vi "36DUT Plot From Spread Sheet.vi"(6 "Plot":T1(ring), 7 "No of Rows":i32=10496, 8 "error in (no error)":errorcluster, 10 "Bank":i32(ring) items=["C1", "C2", "C3", "D_C1", "D_C2", "D_C3", "D_B1_C1", "D_B1_C2", "D_B1_C3"], 11 "file path (dialog if empty)":path) -> (0 "error out":errorcluster, 3 "Delta C_Min Plot":dbl[][](graph) caption="(Y) Multi Plot 2")   [LabVIEW 2012]
uses:
  <vilib>/Utility/file.llb/Read From Spreadsheet File (string).vi
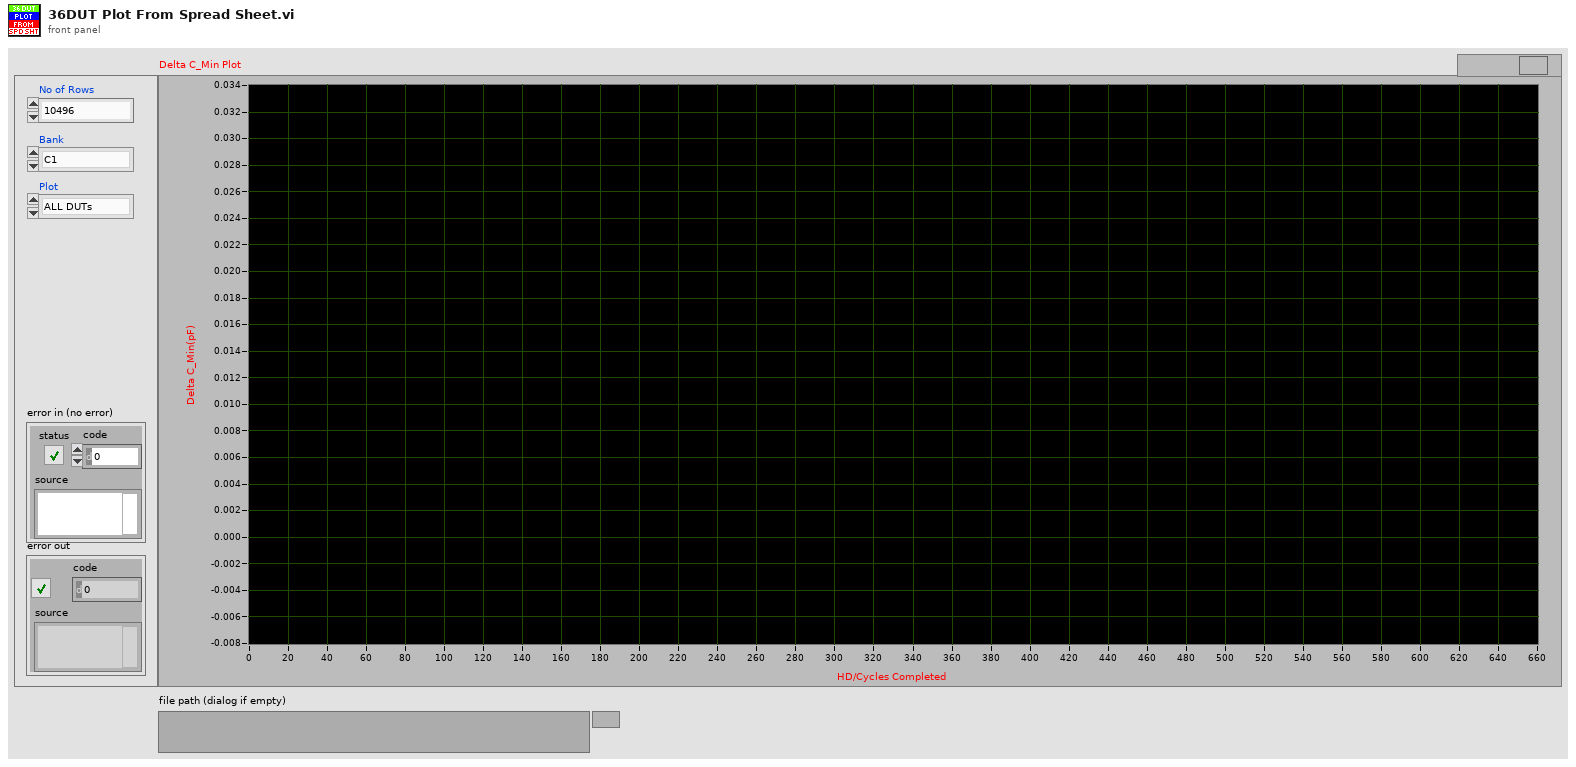
[diagram p1: front panel]
types:
  T1 = enum16{"ALL DUTs", "DUT 01", "DUT 02", "DUT 03", "DUT 04", "DUT 05", "DUT 06", "DUT 07", "DUT 08", "DUT 09", "DUT 10", "DUT 11", "DUT 12", "DUT 13", "DUT 14", "DUT 15", "DUT 16", "DUT 17", "DUT 18", "DUT 19", "DUT 20", "DUT 21", "DUT 22", "DUT 23", "DUT 24", "DUT 25", "DUT 26", "DUT 27", "DUT 28", "DUT 29", "DUT 30", "DUT 31", "DUT 32", "DUT 33", "DUT 34", "DUT 35", "DUT 36"}
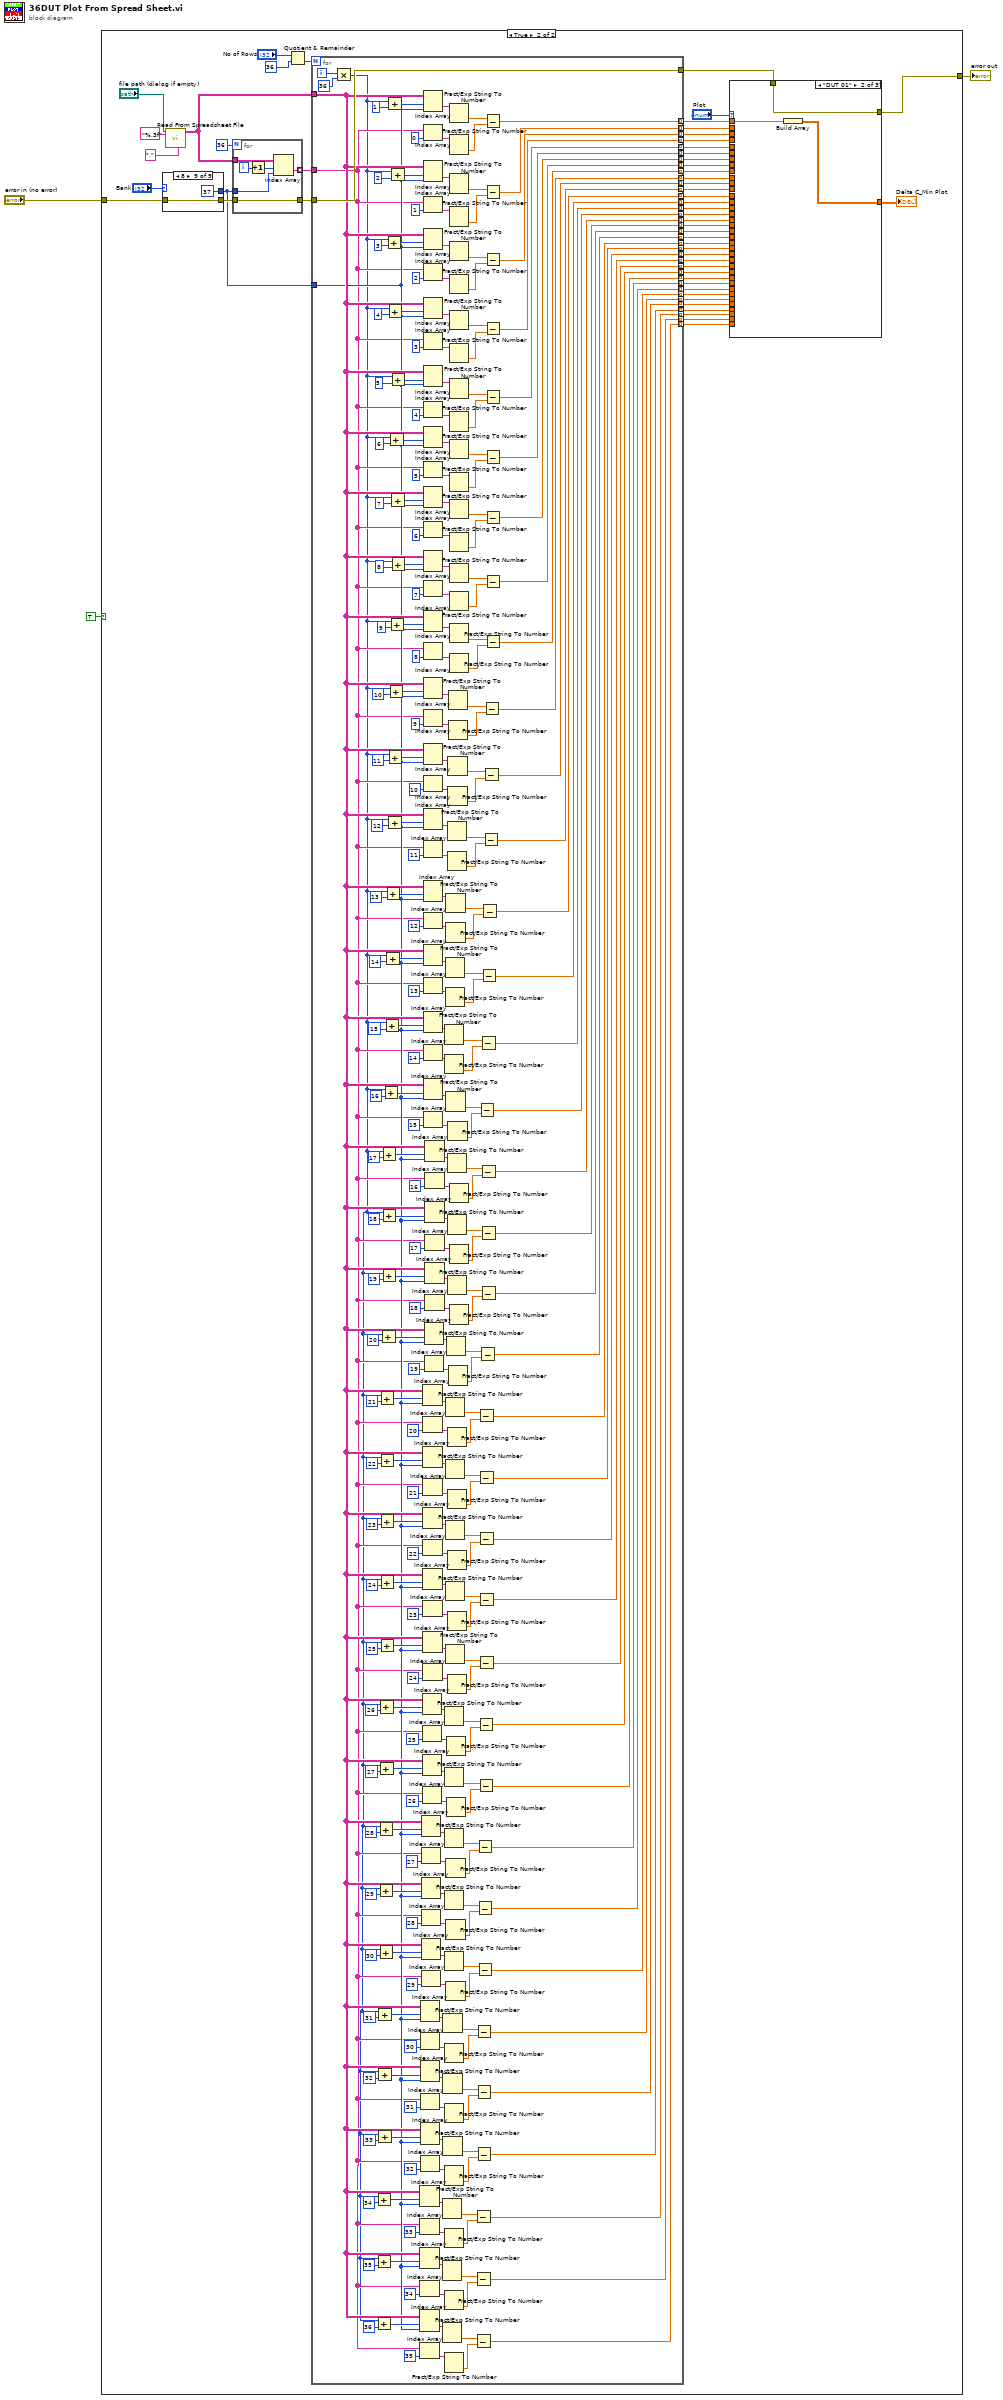
[diagram p0: block diagram]
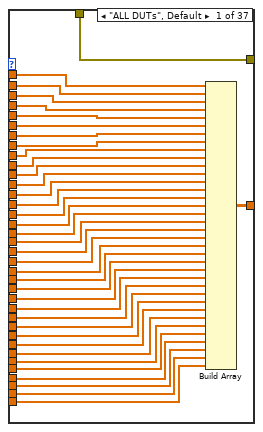
[diagram p3: hidden frame]
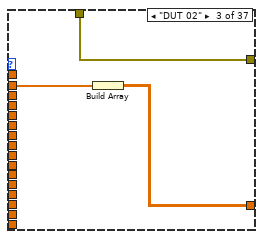
[diagram p4: hidden frame]
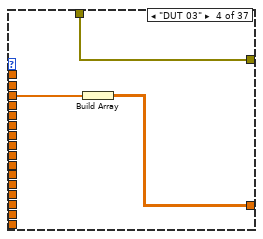
[diagram p5: hidden frame]
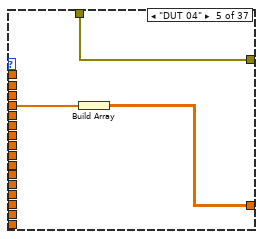
[diagram p6: hidden frame]
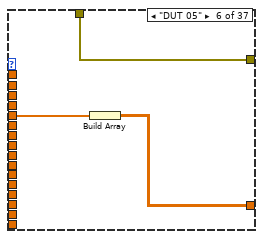
[diagram p7: hidden frame]
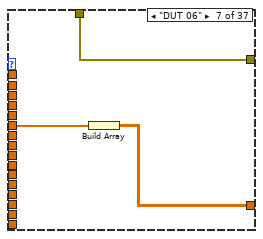
[diagram p8: hidden frame]
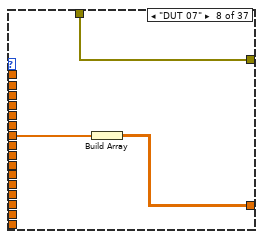
[diagram p9: hidden frame]
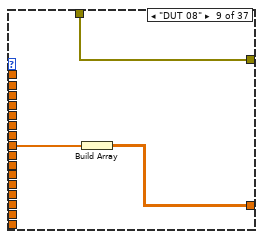
[diagram p10: hidden frame]
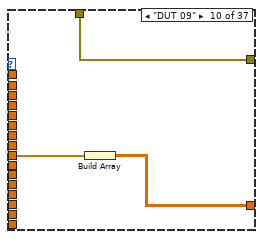
[diagram p11: hidden frame]
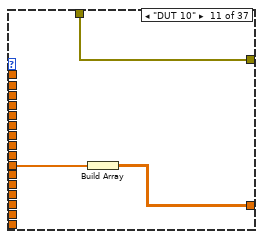
[diagram p12: hidden frame]
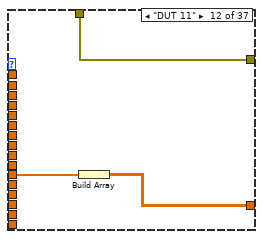
[diagram p13: hidden frame]
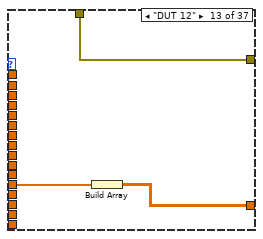
[diagram p14: hidden frame]
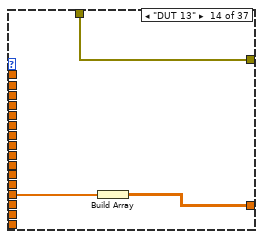
[diagram p15: hidden frame]
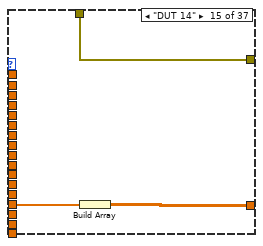
[diagram p16: hidden frame]
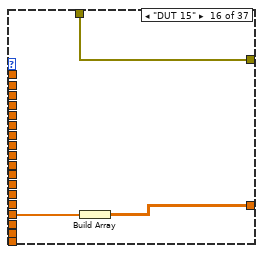
[diagram p17: hidden frame]
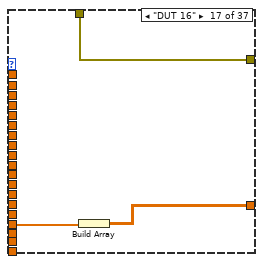
[diagram p18: hidden frame]
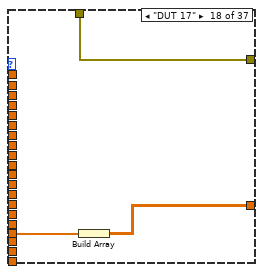
[diagram p19: hidden frame]
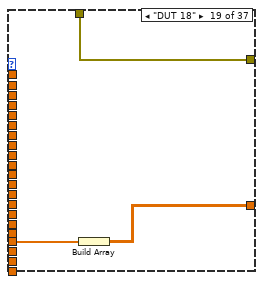
[diagram p20: hidden frame]
diagram:
  n1 = case shown="True" TRUE {
    tunnel: "error in (no error)" -> [w4 w31]
    tunnel: [w4 w25] -> w2
    frame False {
    }
    frame True {
      n2 = case shown="8" "Bank" {
        tunnel: [5 40 75 119 120 121 35 36 37] -> w27
        tunnel: [w205 w207 w209 w212 w214 w216 w217 w219 w221] -> w28
        tunnel: w31 -> [w205 w207 w209 w212 w214 w216 w217 w219 w221]
        frame 0, Default {
        }
        frame 1 {
        }
        frame 2 {
        }
        frame 3 {
        }
        frame 4 {
        }
        frame 5 {
        }
        frame 6 {
        }
        frame 7 {
        }
        frame 8 {
        }
      }
      n3 = call-poly <vilib>:"Read From Spreadsheet File.vi"("delimiter (\\t)"="," ("delimiter (\\t)"), "format (%s)"="%.3f" ("format (%.3f)"), "file path (dialog if empty)"="file path (dialog if empty)") -> ("all rows"=w55:string[][])  [unwired: 4 in, 4 out]
      n4 = for {
        N: 36 -> [_]
        tunnel: w55 -> [w523]
        tunnel: [w522] -> w54 mode=indexing
        tunnel: w27 -> [w518]
        tunnel: [w519] -> w30
        tunnel: w28 -> [w519]
        i -> [w521]
        n5 = Increment(x=w521) -> (x+1=w520:i32)
        n6 = Index Array(array=w523, index (row)=w520, index (col)=w518) -> (element=w522:string)
      }
      n7 = Quotient & Remainder(x="No of Rows", y=36) -> (floor(x/y)=w50:i32)  [unwired: 1 out]
      n8 = for {
        N: w50 -> [_]
        tunnel: w55 -> [w246]
        tunnel: w54 -> [w244]
        tunnel: [w404] -> w48 mode=indexing
        tunnel: [w403] -> w47 mode=indexing
        tunnel: [w402] -> w46 mode=indexing
        tunnel: [w401] -> w45 mode=indexing
        tunnel: [w400] -> w44 mode=indexing
        tunnel: [w399] -> w43 mode=indexing
        tunnel: [w398] -> w42 mode=indexing
        tunnel: [w397] -> w41 mode=indexing
        tunnel: [w396] -> w40 mode=indexing
        tunnel: [w395] -> w39 mode=indexing
        tunnel: [w394] -> w38 mode=indexing
        tunnel: [w393] -> w37 mode=indexing
        tunnel: [w392] -> w36 mode=indexing
        tunnel: [w391] -> w35 mode=indexing
        tunnel: [w390] -> w34 mode=indexing
        tunnel: [w389] -> w33 mode=indexing
        tunnel: w30 -> [w388]
        tunnel: [w388] -> w29
        tunnel: w27 -> [w245]
        tunnel: [w243] -> w24 mode=indexing
        tunnel: [w242] -> w23 mode=indexing
        tunnel: [w241] -> w22 mode=indexing
        tunnel: [w240] -> w21 mode=indexing
        tunnel: [w239] -> w20 mode=indexing
        tunnel: [w238] -> w19 mode=indexing
        tunnel: [w237] -> w18 mode=indexing
        tunnel: [w236] -> w17 mode=indexing
        tunnel: [w235] -> w16 mode=indexing
        tunnel: [w234] -> w15 mode=indexing
        tunnel: [w233] -> w14 mode=indexing
        tunnel: [w232] -> w13 mode=indexing
        tunnel: [w231] -> w12 mode=indexing
        tunnel: [w230] -> w11 mode=indexing
        tunnel: [w229] -> w10 mode=indexing
        tunnel: [w228] -> w9 mode=indexing
        tunnel: [w227] -> w8 mode=indexing
        tunnel: [w226] -> w7 mode=indexing
        tunnel: [w225] -> w6 mode=indexing
        tunnel: [w224] -> w5 mode=indexing
        i -> [w387]
        n9 = Multiply(x=w387, y=36) -> (x*y=w223:i32)
        n10 = Add(x=w223, y=34) -> (x+y=w267:i32)
        n11 = Add(x=w223, y=35) -> (x+y=w254:i32)
        n12 = Add(x=w223, y=36) -> (x+y=w253:i32)
        n13 = Add(x=w223, y=31) -> (x+y=w282:i32)
        n14 = Add(x=w223, y=32) -> (x+y=w281:i32)
        n15 = Add(x=w223, y=33) -> (x+y=w268:i32)
        n16 = Add(x=w223, y=28) -> (x+y=w309:i32)
        n17 = Add(x=w223, y=29) -> (x+y=w296:i32)
        n18 = Add(x=w223, y=30) -> (x+y=w295:i32)
        n19 = Add(x=w223, y=26) -> (x+y=w323:i32)
        n20 = Add(x=w223, y=27) -> (x+y=w310:i32)
        n21 = Add(x=w223, y=21) -> (x+y=w352:i32)
        n22 = Add(x=w223, y=22) -> (x+y=w351:i32)
        n23 = Add(x=w223, y=23) -> (x+y=w338:i32)
        n24 = Add(x=w223, y=24) -> (x+y=w337:i32)
        n25 = Add(x=w223, y=25) -> (x+y=w324:i32)
        n26 = Add(x=w223, y=20) -> (x+y=w365:i32)
        n27 = Add(x=w223, y=17) -> (x+y=w380:i32)
        n28 = Add(x=w223, y=18) -> (x+y=w379:i32)
        n29 = Add(x=w223, y=19) -> (x+y=w366:i32)
        n30 = Add(x=w223, y=16) -> (x+y=w409:i32)
        n31 = Add(x=w223, y=15) -> (x+y=w414:i32)
        n32 = Add(x=w223, y=14) -> (x+y=w423:i32)
        n33 = Add(x=w223, y=13) -> (x+y=w428:i32)
        n34 = Add(x=w223, y=3) -> (x+y=w483:i32)
        n35 = Add(x=w223, y=1) -> (x+y=w505:i32)
        n36 = Add(x=w223, y=12) -> (x+y=w437:i32)
        n37 = Add(x=w223, y=4) -> (x+y=w482:i32)
        n38 = Add(x=w223, y=11) -> (x+y=w442:i32)
        n39 = Add(x=w223, y=10) -> (x+y=w451:i32)
        n40 = Add(x=w223, y=6) -> (x+y=w468:i32)
        n41 = Add(x=w223, y=9) -> (x+y=w498:i32)
        n42 = Add(x=w223, y=2) -> (x+y=w502:i32)
        n43 = Add(x=w223, y=7) -> (x+y=w461:i32)
        n44 = Add(x=w223, y=5) -> (x+y=w475:i32)
        n45 = Add(x=w223, y=8) -> (x+y=w455:i32)
        n46 = Index Array(array=w246, index (row)=w267, index (col)=w245) -> (element=w262:string)
        n47 = Index Array(array=w244, index=33) -> (element=w264:string)
        n48 = Index Array(array=w246, index (row)=w254, index (col)=w245) -> (element=w259:string)
        n49 = Index Array(array=w244, index=34) -> (element=w257:string)
        n50 = Index Array(array=w246, index (row)=w253, index (col)=w245) -> (element=w248:string)
        n51 = Index Array(array=w244, index=35) -> (element=w250:string)
        n52 = Index Array(array=w246, index (row)=w282, index (col)=w245) -> (element=w287:string)
        n53 = Index Array(array=w244, index=30) -> (element=w285:string)
        n54 = Index Array(array=w246, index (row)=w281, index (col)=w245) -> (element=w276:string)
        n55 = Index Array(array=w244, index=31) -> (element=w278:string)
        n56 = Index Array(array=w246, index (row)=w268, index (col)=w245) -> (element=w273:string)
        n57 = Index Array(array=w244, index=32) -> (element=w271:string)
        n58 = Index Array(array=w246, index (row)=w309, index (col)=w245) -> (element=w304:string)
        n59 = Index Array(array=w244, index=27) -> (element=w306:string)
        n60 = Index Array(array=w246, index (row)=w296, index (col)=w245) -> (element=w301:string)
        n61 = Index Array(array=w244, index=28) -> (element=w299:string)
        n62 = Index Array(array=w246, index (row)=w295, index (col)=w245) -> (element=w290:string)
        n63 = Index Array(array=w244, index=29) -> (element=w292:string)
        n64 = Index Array(array=w246, index (row)=w323, index (col)=w245) -> (element=w318:string)
        n65 = Index Array(array=w244, index=25) -> (element=w320:string)
        n66 = Index Array(array=w246, index (row)=w310, index (col)=w245) -> (element=w315:string)
        n67 = Index Array(array=w244, index=26) -> (element=w313:string)
        n68 = Index Array(array=w246, index (row)=w352, index (col)=w245) -> (element=w357:string)
        n69 = Index Array(array=w244, index=20) -> (element=w355:string)
        n70 = Index Array(array=w246, index (row)=w351, index (col)=w245) -> (element=w346:string)
        n71 = Index Array(array=w244, index=21) -> (element=w348:string)
        n72 = Index Array(array=w246, index (row)=w338, index (col)=w245) -> (element=w343:string)
        n73 = Index Array(array=w244, index=22) -> (element=w341:string)
        n74 = Index Array(array=w246, index (row)=w337, index (col)=w245) -> (element=w332:string)
        n75 = Index Array(array=w244, index=23) -> (element=w334:string)
        n76 = Index Array(array=w246, index (row)=w324, index (col)=w245) -> (element=w329:string)
        n77 = Index Array(array=w244, index=24) -> (element=w327:string)
        n78 = Index Array(array=w246, index (row)=w505, index (col)=w245) -> (element=w516:string)
        n79 = Index Array(array=w244, index=0) -> (element=w514:string)
        n80 = Index Array(array=w246, index (row)=w502, index (col)=w245) -> (element=w507:string)
        n81 = Index Array(array=w244, index=1) -> (element=w509:string)
        n82 = Index Array(array=w246, index (row)=w483, index (col)=w245) -> (element=w495:string)
        n83 = Index Array(array=w244, index=2) -> (element=w493:string)
        n84 = Index Array(array=w246, index (row)=w482, index (col)=w245) -> (element=w485:string)
        n85 = Index Array(array=w244, index=3) -> (element=w487:string)
        n86 = Index Array(array=w246, index (row)=w475, index (col)=w245) -> (element=w481:string)
        n87 = Index Array(array=w244, index=4) -> (element=w479:string)
        n88 = Index Array(array=w246, index (row)=w468, index (col)=w245) -> (element=w470:string)
        n89 = Index Array(array=w244, index=5) -> (element=w472:string)
        n90 = Index Array(array=w246, index (row)=w461, index (col)=w245) -> (element=w467:string)
        n91 = Index Array(array=w244, index=6) -> (element=w465:string)
        n92 = Index Array(array=w246, index (row)=w455, index (col)=w245) -> (element=w454:string)
        n93 = Index Array(array=w244, index=7) -> (element=w458:string)
        n94 = Index Array(array=w246, index (row)=w498, index (col)=w245) -> (element=w501:string)
        n95 = Index Array(array=w244, index=8) -> (element=w499:string)
        n96 = Index Array(array=w246, index (row)=w451, index (col)=w245) -> (element=w448:string)
        n97 = Index Array(array=w244, index=9) -> (element=w450:string)
        n98 = Index Array(array=w246, index (row)=w442, index (col)=w245) -> (element=w445:string)
        n99 = Index Array(array=w244, index=10) -> (element=w443:string)
        n100 = Index Array(array=w246, index (row)=w437, index (col)=w245) -> (element=w434:string)
        n101 = Index Array(array=w244, index=11) -> (element=w436:string)
        n102 = Index Array(array=w246, index (row)=w428, index (col)=w245) -> (element=w431:string)
        n103 = Index Array(array=w244, index=12) -> (element=w429:string)
        n104 = Index Array(array=w246, index (row)=w423, index (col)=w245) -> (element=w420:string)
        n105 = Index Array(array=w244, index=13) -> (element=w422:string)
        n106 = Index Array(array=w246, index (row)=w414, index (col)=w245) -> (element=w417:string)
        n107 = Index Array(array=w244, index=14) -> (element=w415:string)
        n108 = Index Array(array=w246, index (row)=w409, index (col)=w245) -> (element=w406:string)
        n109 = Index Array(array=w244, index=15) -> (element=w408:string)
        n110 = Index Array(array=w246, index (row)=w365, index (col)=w245) -> (element=w360:string)
        n111 = Index Array(array=w244, index=19) -> (element=w362:string)
        n112 = Index Array(array=w246, index (row)=w380, index (col)=w245) -> (element=w385:string)
        n113 = Index Array(array=w244, index=16) -> (element=w383:string)
        n114 = Index Array(array=w246, index (row)=w379, index (col)=w245) -> (element=w374:string)
        n115 = Index Array(array=w244, index=17) -> (element=w376:string)
        n116 = Index Array(array=w246, index (row)=w366, index (col)=w245) -> (element=w371:string)
        n117 = Index Array(array=w244, index=18) -> (element=w369:string)
        n118 = Fract/Exp String To Number(string=w262) -> (number=w265:dbl)  [unwired: 3 in, 1 out]
        n119 = Fract/Exp String To Number(string=w259) -> (number=w256:dbl)  [unwired: 3 in, 1 out]
        n120 = Fract/Exp String To Number(string=w248) -> (number=w251:dbl)  [unwired: 3 in, 1 out]
        n121 = Fract/Exp String To Number(string=w287) -> (number=w284:dbl)  [unwired: 3 in, 1 out]
        n122 = Fract/Exp String To Number(string=w276) -> (number=w279:dbl)  [unwired: 3 in, 1 out]
        n123 = Fract/Exp String To Number(string=w273) -> (number=w270:dbl)  [unwired: 3 in, 1 out]
        n124 = Fract/Exp String To Number(string=w304) -> (number=w307:dbl)  [unwired: 3 in, 1 out]
        n125 = Fract/Exp String To Number(string=w301) -> (number=w298:dbl)  [unwired: 3 in, 1 out]
        n126 = Fract/Exp String To Number(string=w290) -> (number=w293:dbl)  [unwired: 3 in, 1 out]
        n127 = Fract/Exp String To Number(string=w264) -> (number=w266:dbl)  [unwired: 3 in, 1 out]
        n128 = Fract/Exp String To Number(string=w257) -> (number=w255:dbl)  [unwired: 3 in, 1 out]
        n129 = Fract/Exp String To Number(string=w250) -> (number=w252:dbl)  [unwired: 3 in, 1 out]
        n130 = Fract/Exp String To Number(string=w417) -> (number=w413:dbl)  [unwired: 3 in, 1 out]
        n131 = Fract/Exp String To Number(string=w415) -> (number=w412:dbl)  [unwired: 3 in, 1 out]
        n132 = Fract/Exp String To Number(string=w318) -> (number=w321:dbl)  [unwired: 3 in, 1 out]
        n133 = Fract/Exp String To Number(string=w315) -> (number=w312:dbl)  [unwired: 3 in, 1 out]
        n134 = Fract/Exp String To Number(string=w285) -> (number=w283:dbl)  [unwired: 3 in, 1 out]
        n135 = Fract/Exp String To Number(string=w278) -> (number=w280:dbl)  [unwired: 3 in, 1 out]
        n136 = Fract/Exp String To Number(string=w271) -> (number=w269:dbl)  [unwired: 3 in, 1 out]
        n137 = Fract/Exp String To Number(string=w420) -> (number=w424:dbl)  [unwired: 3 in, 1 out]
        n138 = Fract/Exp String To Number(string=w422) -> (number=w425:dbl)  [unwired: 3 in, 1 out]
        n139 = Fract/Exp String To Number(string=w357) -> (number=w354:dbl)  [unwired: 3 in, 1 out]
        n140 = Fract/Exp String To Number(string=w346) -> (number=w349:dbl)  [unwired: 3 in, 1 out]
        n141 = Fract/Exp String To Number(string=w343) -> (number=w340:dbl)  [unwired: 3 in, 1 out]
        n142 = Fract/Exp String To Number(string=w332) -> (number=w335:dbl)  [unwired: 3 in, 1 out]
        n143 = Fract/Exp String To Number(string=w329) -> (number=w326:dbl)  [unwired: 3 in, 1 out]
        n144 = Fract/Exp String To Number(string=w431) -> (number=w427:dbl)  [unwired: 3 in, 1 out]
        n145 = Fract/Exp String To Number(string=w429) -> (number=w426:dbl)  [unwired: 3 in, 1 out]
        n146 = Fract/Exp String To Number(string=w406) -> (number=w410:dbl)  [unwired: 3 in, 1 out]
        n147 = Fract/Exp String To Number(string=w306) -> (number=w308:dbl)  [unwired: 3 in, 1 out]
        n148 = Fract/Exp String To Number(string=w299) -> (number=w297:dbl)  [unwired: 3 in, 1 out]
        n149 = Fract/Exp String To Number(string=w292) -> (number=w294:dbl)  [unwired: 3 in, 1 out]
        n150 = Fract/Exp String To Number(string=w360) -> (number=w363:dbl)  [unwired: 3 in, 1 out]
        n151 = Fract/Exp String To Number(string=w320) -> (number=w322:dbl)  [unwired: 3 in, 1 out]
        n152 = Fract/Exp String To Number(string=w313) -> (number=w311:dbl)  [unwired: 3 in, 1 out]
        n153 = Fract/Exp String To Number(string=w434) -> (number=w438:dbl)  [unwired: 3 in, 1 out]
        n154 = Fract/Exp String To Number(string=w436) -> (number=w439:dbl)  [unwired: 3 in, 1 out]
        n155 = Fract/Exp String To Number(string=w385) -> (number=w382:dbl)  [unwired: 3 in, 1 out]
        n156 = Fract/Exp String To Number(string=w374) -> (number=w377:dbl)  [unwired: 3 in, 1 out]
        n157 = Fract/Exp String To Number(string=w371) -> (number=w368:dbl)  [unwired: 3 in, 1 out]
        n158 = Fract/Exp String To Number(string=w355) -> (number=w353:dbl)  [unwired: 3 in, 1 out]
        n159 = Fract/Exp String To Number(string=w348) -> (number=w350:dbl)  [unwired: 3 in, 1 out]
        n160 = Fract/Exp String To Number(string=w341) -> (number=w339:dbl)  [unwired: 3 in, 1 out]
        n161 = Fract/Exp String To Number(string=w334) -> (number=w336:dbl)  [unwired: 3 in, 1 out]
        n162 = Fract/Exp String To Number(string=w327) -> (number=w325:dbl)  [unwired: 3 in, 1 out]
        n163 = Fract/Exp String To Number(string=w445) -> (number=w441:dbl)  [unwired: 3 in, 1 out]
        n164 = Fract/Exp String To Number(string=w443) -> (number=w440:dbl)  [unwired: 3 in, 1 out]
        n165 = Fract/Exp String To Number(string=w408) -> (number=w411:dbl)  [unwired: 3 in, 1 out]
        n166 = Fract/Exp String To Number(string=w448) -> (number=w452:dbl)  [unwired: 3 in, 1 out]
        n167 = Fract/Exp String To Number(string=w450) -> (number=w453:dbl)  [unwired: 3 in, 1 out]
        n168 = Fract/Exp String To Number(string=w362) -> (number=w364:dbl)  [unwired: 3 in, 1 out]
        n169 = Fract/Exp String To Number(string=w383) -> (number=w381:dbl)  [unwired: 3 in, 1 out]
        n170 = Fract/Exp String To Number(string=w376) -> (number=w378:dbl)  [unwired: 3 in, 1 out]
        n171 = Fract/Exp String To Number(string=w369) -> (number=w367:dbl)  [unwired: 3 in, 1 out]
        n172 = Fract/Exp String To Number(string=w516) -> (number=w513:dbl)  [unwired: 3 in, 1 out]
        n173 = Fract/Exp String To Number(string=w514) -> (number=w512:dbl)  [unwired: 3 in, 1 out]
        n174 = Fract/Exp String To Number(string=w507) -> (number=w510:dbl)  [unwired: 3 in, 1 out]
        n175 = Fract/Exp String To Number(string=w509) -> (number=w511:dbl)  [unwired: 3 in, 1 out]
        n176 = Fract/Exp String To Number(string=w495) -> (number=w492:dbl)  [unwired: 3 in, 1 out]
        n177 = Fract/Exp String To Number(string=w493) -> (number=w491:dbl)  [unwired: 3 in, 1 out]
        n178 = Fract/Exp String To Number(string=w485) -> (number=w488:dbl)  [unwired: 3 in, 1 out]
        n179 = Fract/Exp String To Number(string=w487) -> (number=w489:dbl)  [unwired: 3 in, 1 out]
        n180 = Fract/Exp String To Number(string=w481) -> (number=w478:dbl)  [unwired: 3 in, 1 out]
        n181 = Fract/Exp String To Number(string=w479) -> (number=w477:dbl)  [unwired: 3 in, 1 out]
        n182 = Fract/Exp String To Number(string=w470) -> (number=w473:dbl)  [unwired: 3 in, 1 out]
        n183 = Fract/Exp String To Number(string=w472) -> (number=w474:dbl)  [unwired: 3 in, 1 out]
        n184 = Fract/Exp String To Number(string=w467) -> (number=w464:dbl)  [unwired: 3 in, 1 out]
        n185 = Fract/Exp String To Number(string=w465) -> (number=w463:dbl)  [unwired: 3 in, 1 out]
        n186 = Fract/Exp String To Number(string=w454) -> (number=w459:dbl)  [unwired: 3 in, 1 out]
        n187 = Fract/Exp String To Number(string=w458) -> (number=w460:dbl)  [unwired: 3 in, 1 out]
        n188 = Fract/Exp String To Number(string=w501) -> (number=w497:dbl)  [unwired: 3 in, 1 out]
        n189 = Fract/Exp String To Number(string=w499) -> (number=w496:dbl)  [unwired: 3 in, 1 out]
        n190 = Subtract(x=w265, y=w266) -> (x-y=w226:dbl)
        n191 = Subtract(x=w256, y=w255) -> (x-y=w225:dbl)
        n192 = Subtract(x=w251, y=w252) -> (x-y=w224:dbl)
        n193 = Subtract(x=w284, y=w283) -> (x-y=w229:dbl)
        n194 = Subtract(x=w279, y=w280) -> (x-y=w228:dbl)
        n195 = Subtract(x=w270, y=w269) -> (x-y=w227:dbl)
        n196 = Subtract(x=w307, y=w308) -> (x-y=w232:dbl)
        n197 = Subtract(x=w298, y=w297) -> (x-y=w231:dbl)
        n198 = Subtract(x=w293, y=w294) -> (x-y=w230:dbl)
        n199 = Subtract(x=w321, y=w322) -> (x-y=w234:dbl)
        n200 = Subtract(x=w312, y=w311) -> (x-y=w233:dbl)
        n201 = Subtract(x=w354, y=w353) -> (x-y=w239:dbl)
        n202 = Subtract(x=w349, y=w350) -> (x-y=w238:dbl)
        n203 = Subtract(x=w340, y=w339) -> (x-y=w237:dbl)
        n204 = Subtract(x=w335, y=w336) -> (x-y=w236:dbl)
        n205 = Subtract(x=w326, y=w325) -> (x-y=w235:dbl)
        n206 = Subtract(x=w410, y=w411) -> (x-y=w389:dbl)
        n207 = Subtract(x=w363, y=w364) -> (x-y=w240:dbl)
        n208 = Subtract(x=w413, y=w412) -> (x-y=w390:dbl)
        n209 = Subtract(x=w382, y=w381) -> (x-y=w243:dbl)
        n210 = Subtract(x=w377, y=w378) -> (x-y=w242:dbl)
        n211 = Subtract(x=w368, y=w367) -> (x-y=w241:dbl)
        n212 = Subtract(x=w424, y=w425) -> (x-y=w391:dbl)
        n213 = Subtract(x=w427, y=w426) -> (x-y=w392:dbl)
        n214 = Subtract(x=w438, y=w439) -> (x-y=w393:dbl)
        n215 = Subtract(x=w441, y=w440) -> (x-y=w394:dbl)
        n216 = Subtract(x=w452, y=w453) -> (x-y=w395:dbl)
        n217 = Subtract(x=w513, y=w512) -> (x-y=w404:dbl)
        n218 = Subtract(x=w510, y=w511) -> (x-y=w403:dbl)
        n219 = Subtract(x=w492, y=w491) -> (x-y=w402:dbl)
        n220 = Subtract(x=w488, y=w489) -> (x-y=w401:dbl)
        n221 = Subtract(x=w478, y=w477) -> (x-y=w400:dbl)
        n222 = Subtract(x=w473, y=w474) -> (x-y=w399:dbl)
        n223 = Subtract(x=w464, y=w463) -> (x-y=w398:dbl)
        n224 = Subtract(x=w459, y=w460) -> (x-y=w397:dbl)
        n225 = Subtract(x=w497, y=w496) -> (x-y=w396:dbl)
      }
      n226 = case shown="\"DUT 01\"" "Plot" {
        tunnel: w48 -> [w96 w99 _ _ _ _ _ _ _ _ _ _ _ _ _ _ _ _ _ _ _ _ _ _ _ _ _ _ _ _ _ _ _ _ _ _ _]
        tunnel: w47 -> [w95 _ w101 _ _ _ _ _ _ _ _ _ _ _ _ _ _ _ _ _ _ _ _ _ _ _ _ _ _ _ _ _ _ _ _ _ _]
        tunnel: w46 -> [w94 _ _ w105 _ _ _ _ _ _ _ _ _ _ _ _ _ _ _ _ _ _ _ _ _ _ _ _ _ _ _ _ _ _ _ _ _]
        tunnel: w45 -> [w93 _ _ _ w107 _ _ _ _ _ _ _ _ _ _ _ _ _ _ _ _ _ _ _ _ _ _ _ _ _ _ _ _ _ _ _ _]
        tunnel: w44 -> [w92 _ _ _ _ w111 _ _ _ _ _ _ _ _ _ _ _ _ _ _ _ _ _ _ _ _ _ _ _ _ _ _ _ _ _ _ _]
        tunnel: w43 -> [w91 _ _ _ _ _ w113 _ _ _ _ _ _ _ _ _ _ _ _ _ _ _ _ _ _ _ _ _ _ _ _ _ _ _ _ _ _]
        tunnel: w42 -> [w90 _ _ _ _ _ _ w116 _ _ _ _ _ _ _ _ _ _ _ _ _ _ _ _ _ _ _ _ _ _ _ _ _ _ _ _ _]
        tunnel: w41 -> [w89 _ _ _ _ _ _ _ w120 _ _ _ _ _ _ _ _ _ _ _ _ _ _ _ _ _ _ _ _ _ _ _ _ _ _ _ _]
        tunnel: w40 -> [w88 _ _ _ _ _ _ _ _ w123 _ _ _ _ _ _ _ _ _ _ _ _ _ _ _ _ _ _ _ _ _ _ _ _ _ _ _]
        tunnel: w39 -> [w87 _ _ _ _ _ _ _ _ _ w126 _ _ _ _ _ _ _ _ _ _ _ _ _ _ _ _ _ _ _ _ _ _ _ _ _ _]
        tunnel: w38 -> [w86 _ _ _ _ _ _ _ _ _ _ w129 _ _ _ _ _ _ _ _ _ _ _ _ _ _ _ _ _ _ _ _ _ _ _ _ _]
        tunnel: w37 -> [w85 _ _ _ _ _ _ _ _ _ _ _ w132 _ _ _ _ _ _ _ _ _ _ _ _ _ _ _ _ _ _ _ _ _ _ _ _]
        tunnel: w36 -> [w84 _ _ _ _ _ _ _ _ _ _ _ _ w135 _ _ _ _ _ _ _ _ _ _ _ _ _ _ _ _ _ _ _ _ _ _ _]
        tunnel: w35 -> [w83 _ _ _ _ _ _ _ _ _ _ _ _ _ w138 _ _ _ _ _ _ _ _ _ _ _ _ _ _ _ _ _ _ _ _ _ _]
        tunnel: w34 -> [w82 _ _ _ _ _ _ _ _ _ _ _ _ _ _ w141 _ _ _ _ _ _ _ _ _ _ _ _ _ _ _ _ _ _ _ _ _]
        tunnel: w33 -> [w81 _ _ _ _ _ _ _ _ _ _ _ _ _ _ _ w143 _ _ _ _ _ _ _ _ _ _ _ _ _ _ _ _ _ _ _ _]
        tunnel: [w80 w98 w102 w104 w108 w110 w114 w117 w119 w122 w125 w128 w131 w134 w137 w140 w144 w147 w150 w153 w156 w159 w162 w165 w168 w171 w174 w177 w180 w183 w186 w189 w192 w195 w198 w201 w204] -> w32
        tunnel: w29 -> [w79 w97 w100 w103 w106 w109 w112 w115 w118 w121 w124 w127 w130 w133 w136 w139 w142 w146 w149 w152 w155 w158 w161 w164 w167 w170 w173 w176 w179 w182 w185 w188 w191 w194 w197 w200 w203]
        tunnel: [w79 w97 w100 w103 w106 w109 w112 w115 w118 w121 w124 w127 w130 w133 w136 w139 w142 w146 w149 w152 w155 w158 w161 w164 w167 w170 w173 w176 w179 w182 w185 w188 w191 w194 w197 w200 w203] -> w25
        tunnel: w24 -> [w78 _ _ _ _ _ _ _ _ _ _ _ _ _ _ _ _ w145 _ _ _ _ _ _ _ _ _ _ _ _ _ _ _ _ _ _ _]
        tunnel: w23 -> [w77 _ _ _ _ _ _ _ _ _ _ _ _ _ _ _ _ _ w148 _ _ _ _ _ _ _ _ _ _ _ _ _ _ _ _ _ _]
        tunnel: w22 -> [w76 _ _ _ _ _ _ _ _ _ _ _ _ _ _ _ _ _ _ w151 _ _ _ _ _ _ _ _ _ _ _ _ _ _ _ _ _]
        tunnel: w21 -> [w75 _ _ _ _ _ _ _ _ _ _ _ _ _ _ _ _ _ _ _ w154 _ _ _ _ _ _ _ _ _ _ _ _ _ _ _ _]
        tunnel: w20 -> [w74 _ _ _ _ _ _ _ _ _ _ _ _ _ _ _ _ _ _ _ _ w157 _ _ _ _ _ _ _ _ _ _ _ _ _ _ _]
        tunnel: w19 -> [w73 _ _ _ _ _ _ _ _ _ _ _ _ _ _ _ _ _ _ _ _ _ w160 _ _ _ _ _ _ _ _ _ _ _ _ _ _]
        tunnel: w18 -> [w72 _ _ _ _ _ _ _ _ _ _ _ _ _ _ _ _ _ _ _ _ _ _ w163 _ _ _ _ _ _ _ _ _ _ _ _ _]
        tunnel: w17 -> [w71 _ _ _ _ _ _ _ _ _ _ _ _ _ _ _ _ _ _ _ _ _ _ _ w166 _ _ _ _ _ _ _ _ _ _ _ _]
        tunnel: w16 -> [w70 _ _ _ _ _ _ _ _ _ _ _ _ _ _ _ _ _ _ _ _ _ _ _ _ w169 _ _ _ _ _ _ _ _ _ _ _]
        tunnel: w15 -> [w69 _ _ _ _ _ _ _ _ _ _ _ _ _ _ _ _ _ _ _ _ _ _ _ _ _ w172 _ _ _ _ _ _ _ _ _ _]
        tunnel: w14 -> [w68 _ _ _ _ _ _ _ _ _ _ _ _ _ _ _ _ _ _ _ _ _ _ _ _ _ _ w175 _ _ _ _ _ _ _ _ _]
        tunnel: w13 -> [w67 _ _ _ _ _ _ _ _ _ _ _ _ _ _ _ _ _ _ _ _ _ _ _ _ _ _ _ w178 _ _ _ _ _ _ _ _]
        tunnel: w12 -> [w66 _ _ _ _ _ _ _ _ _ _ _ _ _ _ _ _ _ _ _ _ _ _ _ _ _ _ _ _ w181 _ _ _ _ _ _ _]
        tunnel: w11 -> [w65 _ _ _ _ _ _ _ _ _ _ _ _ _ _ _ _ _ _ _ _ _ _ _ _ _ _ _ _ _ w184 _ _ _ _ _ _]
        tunnel: w10 -> [w64 _ _ _ _ _ _ _ _ _ _ _ _ _ _ _ _ _ _ _ _ _ _ _ _ _ _ _ _ _ _ w187 _ _ _ _ _]
        tunnel: w9 -> [w63 _ _ _ _ _ _ _ _ _ _ _ _ _ _ _ _ _ _ _ _ _ _ _ _ _ _ _ _ _ _ _ w190 _ _ _ _]
        tunnel: w8 -> [w62 _ _ _ _ _ _ _ _ _ _ _ _ _ _ _ _ _ _ _ _ _ _ _ _ _ _ _ _ _ _ _ _ w193 _ _ _]
        tunnel: w7 -> [w61 _ _ _ _ _ _ _ _ _ _ _ _ _ _ _ _ _ _ _ _ _ _ _ _ _ _ _ _ _ _ _ _ _ w196 _ _]
        tunnel: w6 -> [w60 _ _ _ _ _ _ _ _ _ _ _ _ _ _ _ _ _ _ _ _ _ _ _ _ _ _ _ _ _ _ _ _ _ _ w199 _]
        tunnel: w5 -> [w59 _ _ _ _ _ _ _ _ _ _ _ _ _ _ _ _ _ _ _ _ _ _ _ _ _ _ _ _ _ _ _ _ _ _ _ w202]
        frame "ALL DUTs", Default {
          n227 = Build Array(w96, w95, w94, w93, w92, w91, w90, w89, w88, w87, w86, w85, w84, w83, w82, w81, w78, w77, w76, w75, w74, w73, w72, w71, w70, w69, w68, w67, w66, w65, w64, w63, w62, w61, w60, w59) -> (w80:dbl[][])
        }
        frame "DUT 01" {
          n228 = Build Array(w99) -> (w98:dbl[][])
        }
        frame "DUT 02" {
          n229 = Build Array(w101) -> (w102:dbl[][])
        }
        frame "DUT 03" {
          n230 = Build Array(w105) -> (w104:dbl[][])
        }
        frame "DUT 04" {
          n231 = Build Array(w107) -> (w108:dbl[][])
        }
        frame "DUT 05" {
          n232 = Build Array(w111) -> (w110:dbl[][])
        }
        frame "DUT 06" {
          n233 = Build Array(w113) -> (w114:dbl[][])
        }
        frame "DUT 07" {
          n234 = Build Array(w116) -> (w117:dbl[][])
        }
        frame "DUT 08" {
          n235 = Build Array(w120) -> (w119:dbl[][])
        }
        frame "DUT 09" {
          n236 = Build Array(w123) -> (w122:dbl[][])
        }
        frame "DUT 10" {
          n237 = Build Array(w126) -> (w125:dbl[][])
        }
        frame "DUT 11" {
          n238 = Build Array(w129) -> (w128:dbl[][])
        }
        frame "DUT 12" {
          n239 = Build Array(w132) -> (w131:dbl[][])
        }
        frame "DUT 13" {
          n240 = Build Array(w135) -> (w134:dbl[][])
        }
        frame "DUT 14" {
          n241 = Build Array(w138) -> (w137:dbl[][])
        }
        frame "DUT 15" {
          n242 = Build Array(w141) -> (w140:dbl[][])
        }
        frame "DUT 16" {
          n243 = Build Array(w143) -> (w144:dbl[][])
        }
        frame "DUT 17" {
          n244 = Build Array(w145) -> (w147:dbl[][])
        }
        frame "DUT 18" {
          n245 = Build Array(w148) -> (w150:dbl[][])
        }
        frame "DUT 19" {
          n246 = Build Array(w151) -> (w153:dbl[][])
        }
        frame "DUT 20" {
          n247 = Build Array(w154) -> (w156:dbl[][])
        }
        frame "DUT 21" {
          n248 = Build Array(w157) -> (w159:dbl[][])
        }
        frame "DUT 22" {
          n249 = Build Array(w160) -> (w162:dbl[][])
        }
        frame "DUT 23" {
          n250 = Build Array(w163) -> (w165:dbl[][])
        }
        frame "DUT 24" {
          n251 = Build Array(w166) -> (w168:dbl[][])
        }
        frame "DUT 25" {
          n252 = Build Array(w169) -> (w171:dbl[][])
        }
        frame "DUT 26" {
          n253 = Build Array(w172) -> (w174:dbl[][])
        }
        frame "DUT 27" {
          n254 = Build Array(w175) -> (w177:dbl[][])
        }
        frame "DUT 28" {
          n255 = Build Array(w178) -> (w180:dbl[][])
        }
        frame "DUT 29" {
          n256 = Build Array(w181) -> (w183:dbl[][])
        }
        frame "DUT 30" {
          n257 = Build Array(w184) -> (w186:dbl[][])
        }
        frame "DUT 31" {
          n258 = Build Array(w187) -> (w189:dbl[][])
        }
        frame "DUT 32" {
          n259 = Build Array(w190) -> (w192:dbl[][])
        }
        frame "DUT 33" {
          n260 = Build Array(w193) -> (w195:dbl[][])
        }
        frame "DUT 34" {
          n261 = Build Array(w196) -> (w198:dbl[][])
        }
        frame "DUT 35" {
          n262 = Build Array(w199) -> (w201:dbl[][])
        }
        frame "DUT 36" {
          n263 = Build Array(w202) -> (w204:dbl[][])
        }
      }
      "Delta C_Min Plot" <- w32
    }
  }
  "error out" <- w2
